vi "getLineData.vi"(0 "index":i32, 1 "length":i32, 5 "meta":T1={"DYB_Order"=2, "Spalte"=2, "Zeile"=260, "Abstand Datenpunkte"=5.757235038420917e+29, "Abstand Scanzeilen"=-5.4779473692595377e+23, "x-Koordinate 1. Punkt"=3.18299368645e-313, "y-Koordinate 2. Punkt"=0.007812501473381417, "Neigungswinkel Scanfeld"=8.487983164e-314, "Einheit Variablen"=2, "stepVal"=0.0, "stepValNum"=0.0, "offsetVal"=0.0, "unitVal"=2}, 7 "frameNO":i32, 9 "data":i32[](array[numeric]), 11 "error in":T2) -> (4 "linearray":sgl[](array[numeric]), 6 "Unit value":string, 15 "error out":T2)   [LabVIEW 2016]
doc: "Processes data from the LineView passed by the input \"data\". This VI is part of the VI getDataLine.vi. We recommend to use getDataLine.vi to access data from the lineVIEW instead of this one.\nThe inputs are\n- Length: number of the datapoints in the input \"array\"\n- Index: index of the newest data point\n- Meta: meta data to process the raw data\n- frameNO: Number of frames that have already been processed\n- data: array with raw data points\nThe outputs are:\n- Linearray: array that contains the processed LineView-data. The newest data point has always the highest index in this array\n- Unit value: Unit of depended variable\n- Unit xy: Unit of independent variable"
uses:
  Controls/Error_Out.ctl
  Controls/Metadata-Cluster.ctl
  Files_ASC500/DLL/ASC500_RemoteControlV27.dll
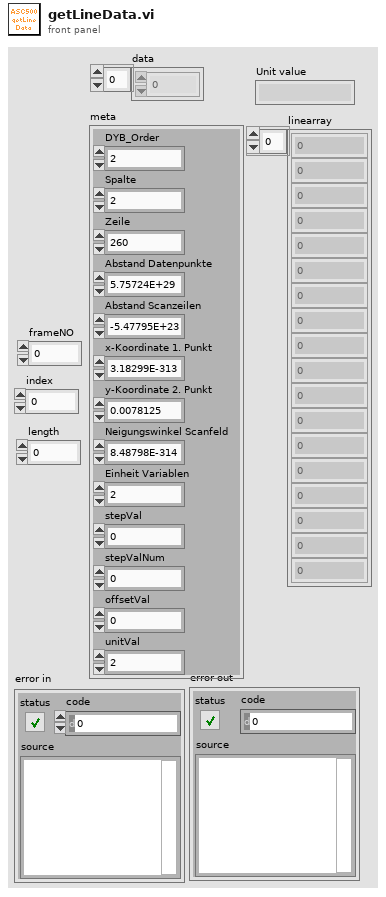
[diagram p1: front panel]
types:
  T1 = typedef "Metadata-Cluster.ctl" = cluster{"DYB_Order":i32, "Spalte":i32, "Zeile":i32, "Abstand Datenpunkte":dbl, "Abstand Scanzeilen":dbl, "x-Koordinate 1. Punkt":dbl, "y-Koordinate 2. Punkt":dbl, "Neigungswinkel Scanfeld":dbl, "Einheit Variablen":i32, "stepVal":dbl, "stepValNum":dbl, "offsetVal":dbl, "unitVal":i32}
  T2 = typedef "Error_Out.ctl" = errorcluster
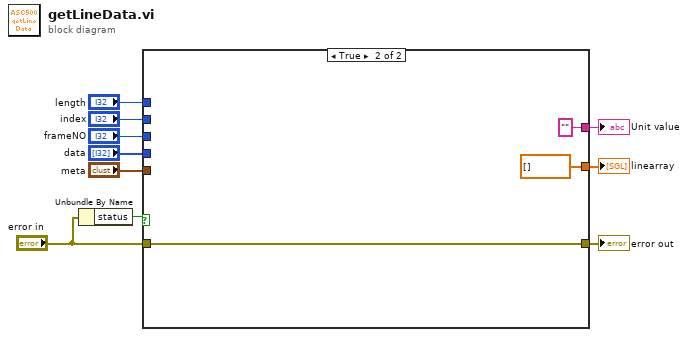
[diagram p0: block diagram]
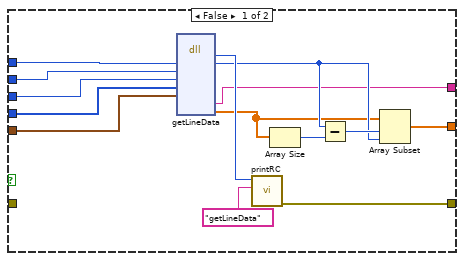
[diagram p2: hidden frame]
diagram:
  n1 = Unbundle By Name("error in") -> ("status"=w8:bool)
  n2 = case shown="True" w8 {
    tunnel: "error in" -> [_ w27]
    tunnel: [w23 w27] -> w9
    tunnel: "index" -> [w14 _]
    tunnel: [w17 sgl[] [] ("value_out 2")] -> w6
    tunnel: "length" -> [w16 _]
    tunnel: "data" -> [w15 _]
    tunnel: "frameNO" -> [w13 _]
    tunnel: "meta" -> [w12 _]
    tunnel: [w11 "" ("Unit value")] -> w1
    frame False {
      n3 = dll-call lib="G:/SCMOperations/Share/ELE/Produkt Information/ASC500/04 Remote Control/02 development versions/2018Nov06/Files_ASC500/DLL/ASC500_RemoteControlV27.dll" fn="getLineData"("length"=w16, "index"=w14, "frameNO"=w13, "data"=w15, "meta"=w12) -> ("RC"=w22:u32, "length"=w19:i32, "Unit value"=w11:string, "linearray"=w18:sgl[])  [unwired: 9 in, 2 out]
      n4 = call "printRC.vi"("additional information"="getLineData", "RC"=w22) -> ("error out"=w23:T2)  [unwired: 9 in]
      n5 = Array Size(array=w18) -> (size(s)=w21:i32)
      n6 = Subtract(x=w19, y=w21) -> (x-y=w20:i32)
      n7 = Array Subset(array=w18, index=w20, length=w19) -> (w17:sgl[])
    }
    frame True {
    }
  }
  "error out" <- w9
  "linearray" <- w6
  "Unit value" <- w1
